vi "set_voltages.vi"(4 "Vmax_z":dbl, 6 "Vmin_z":dbl, 8 "error in (no error)":errorcluster, 9 "Vmax_y":dbl, 10 "Vmin_y":dbl, 11 "ImagingModeDL090130Frame in":refnum<class "ImagingModeDL090130Frame.lvclass">) -> (0 "error out":errorcluster, 3 "ImagingModeDL090130Frame out":refnum<class "ImagingModeDL090130Frame.lvclass">)   [LabVIEW 2010, in "ImagingModeDL090130Frame.lvclass"]
uses:
  ImagingModeDL090130Frame.lvclass
  ImagingModeDL090130Frame.lvclass/ImagingModeDL090130Frame.ctl
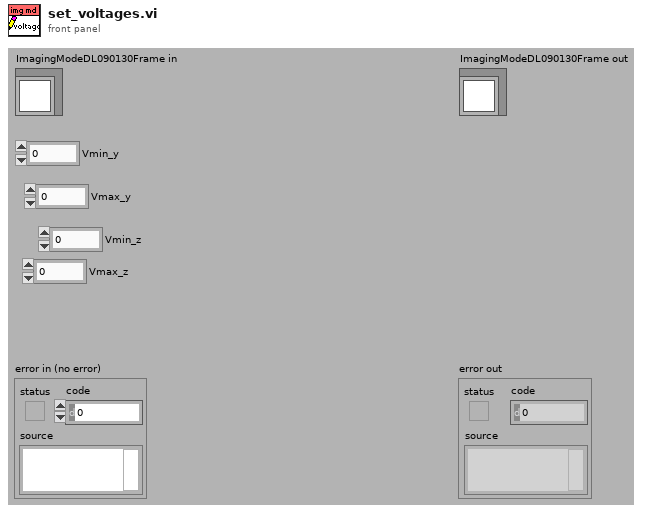
[diagram p1: front panel]
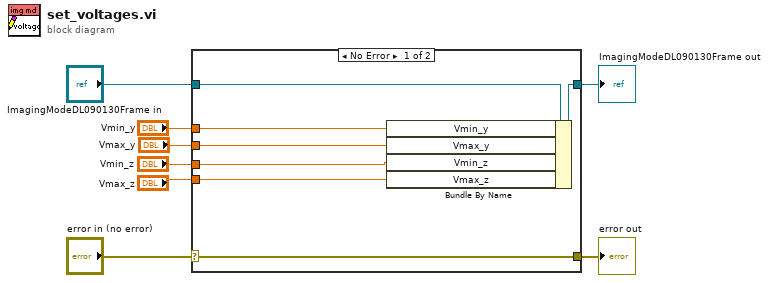
[diagram p0: block diagram]
diagram:
  n1 = case shown="No Error" "error in (no error)" {
    selector: "error in (no error)" -> [w15 w16]
    tunnel: [w15 w16] -> w7
    tunnel: [w13 w17] -> w5
    tunnel: "ImagingModeDL090130Frame in" -> [w14 w17]
    tunnel: "Vmin_y" -> [w12 _]
    tunnel: "Vmax_y" -> [w11 _]
    tunnel: "Vmin_z" -> [w10 _]
    tunnel: "Vmax_z" -> [w9 _]
    frame No Error {
      n2 = Bundle By Name(cluster=w14, "Vmin_y"=w12, "Vmax_y"=w11, "Vmin_z"=w10, "Vmax_z"=w9) -> (w13:refnum<class "ImagingModeDL090130Frame.lvclass">)
    }
    frame Error {
    }
  }
  "error out" <- w7
  "ImagingModeDL090130Frame out" <- w5
